vi "ReadReply_Full.vi"(8 "error in (no error)":errorcluster, 9 "timeout ms (60000)":i32=60000, 11 "TCP in":refnum<k5>) -> (0 "error out":errorcluster, 2 "Info":T1, 3 "TCP out":refnum<k5>)   [LabVIEW 2019]
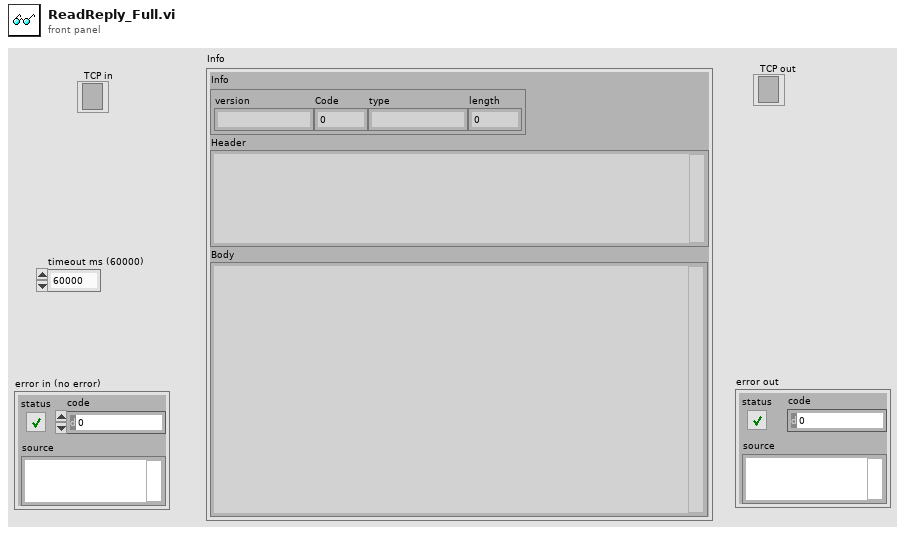
[diagram p1: front panel]
types:
  T1 = cluster{"Info":cluster{"version":string, "Code":i32, "type":string, "length":i32}, "Header":string, "Body":string}
  T2 = cluster{string, "default value 2":i32, "value":string, i32}
  T3 = cluster{cluster{string, "default value 2":i32, "value":string, i32}, "String":string, "String":string}
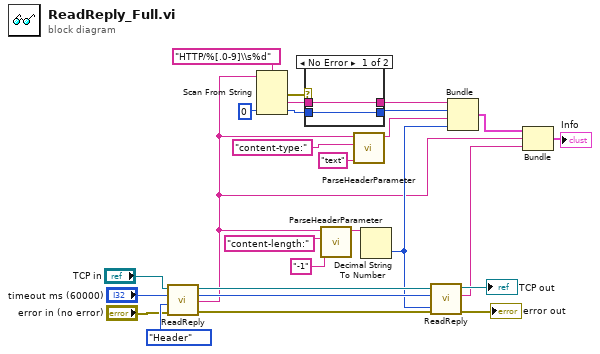
[diagram p0: block diagram]
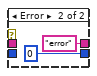
[diagram p2: hidden frame]
diagram:
  n1 = call "ReadReply.vi"("error in (no error)"="error in (no error)", "Type"=enum16{"Header", "Body"}."Header", "timeout ms (60000)"="timeout ms (60000)", "TCP in"="TCP in") -> ("error out"=w19:errorcluster, "String"=w7:string, "TCP out"=w20:refnum<k5>)  [unwired: 5 in]
  n2 = Scan From String(format string="HTTP/%[.0-9]\\s%d", input string=w7, default 2=0 ("default value 2")) -> (error out=w5:errorcluster, output 1=w3:string, output 2=w1:i32)  [unwired: 3 in, 2 out]
  n3 = case shown="No Error" w5 {
    tunnel: [w28 "error"] -> w4
    tunnel: w3 -> [w28 _]
    tunnel: [w27 0 ("default value 2")] -> w2
    tunnel: w1 -> [w27 _]
    frame No Error {
    }
    frame Error {
    }
  }
  n4 = call "ParseHeaderParameter.vi"("default value"="-1", "property"="content-length:" ("regular expression"), "header"=w7) -> ("value"=w9:string)  [unwired: 8 in]
  n5 = call "ParseHeaderParameter.vi"("default value"="text" ("trimmed string"), "property"="content-type:" ("regular expression"), "header"=w7) -> ("value"=w13:string)  [unwired: 8 in]
  n6 = Decimal String To Number(string=w9) -> (number=w8:i32)  [unwired: 2 in, 1 out]
  n7 = call "ReadReply.vi"("length"=w8, "error in (no error)"=w19, "timeout ms (60000)"="timeout ms (60000)", "TCP in"=w20) -> ("error out"=→"error out":errorcluster, "String"=w16:string, "TCP out"=→"TCP out":refnum<k5>)  [unwired: 5 in]
  n8 = Bundle(w4, "default value 2"=w2, "value"=w13, w8) -> (w15:T2)  [unwired: 1 in]
  n9 = Bundle(w15, "String"=w7, "String"=w16) -> (→"Info":T3)  [unwired: 1 in]
